vi "TreeSelectBratCallback.vi"(4 "Glyph Indices":T1, 5 "Event Data":T3, 6 "Tree Ref":refnum<vi>, 7 "Event Common Data":cluster{"Source":T4, "Type":T5, "Time":u32} {"Source" items=["LabVIEW UI"=0, "ActiveX"=1, "User Event"=25]}) -> ()   [LabVIEW 2012]
uses:
  <vilib>/event_ctls.llb/eventsource.ctl
  <vilib>/event_ctls.llb/lveventtype.ctl
  <vilib>/Utility/miscctls.llb/LVPoint32TypeDef.ctl
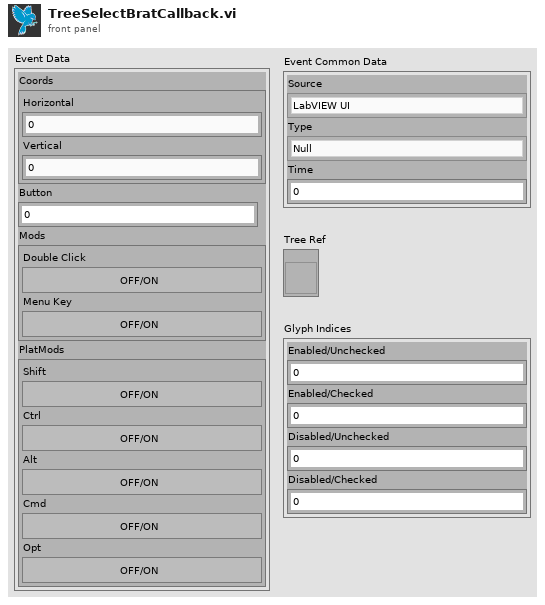
[diagram p1: front panel]
types:
  T1 = cluster{"Enabled/Unchecked":i32, "Enabled/Checked":i32, "Disabled/Unchecked":i32, "Disabled/Checked":i32}
  T2 = typedef "LVPoint32TypeDef.ctl" = cluster{"Horizontal":i32, "Vertical":i32}
  T3 = cluster{"Coords":T2, "Button":u16, "Mods":cluster{"Double Click":bool, "Menu Key":bool}, "PlatMods":cluster{"Shift":bool, "Ctrl":bool, "Alt":bool, "Cmd":bool, "Opt":bool}}
  T4 = typedef "eventsource.ctl" = u32
  T5 = typedef "lveventtype.ctl" = enum32{"Null", "Timeout", "Annotation Menu Selection", "Annotation Menu Selection?", "App Instance Close", "App Instance Close?", "Autoscale Range Change", "Cell Edit", "Cell Edit?", "Cursor Grab", "Cursor Grab?", "Cursor Menu Selection", "Cursor Menu Selection?", "Cursor Move", "Cursor Release", "Data Change", "Direction Change", "Display State Change", "Drag Ended", "Drag Enter", "Drag Leave", "Drag Over", "Drag Source Update", "Drag Starting", "Drag Starting?", "Drop", "Exec State Change", "Key Down", "Key Down?", "Key Repeat", "Key Repeat?", "Key Up", "Listbox Double Click", "Menu Activation?", "Menu Selection (App)", "Menu Selection? (App)", "Menu Selection (User)", "Mouse Down", "Mouse Down?", "Mouse Enter", "Mouse Leave", "Mouse Move", "Mouse Up", "NI Security User Change (App)", "Pane Size", "Panel Close", "Panel Close?", "Panel Resize", "Plot Attribute Change", "Scale Range Change", "Shortcut Menu Activation?", "Shortcut Menu Selection (App)", "Shortcut Menu Selection? (App)", "Shortcut Menu Selection (User)", "Tree Double Click", "Tree Drag", "Tree Drag?", "Tree Drop", "Tree Drop?", "Tree Item Close", "Tree Item Close?", "Tree Item Open", "Tree Item Open?", "Value Change"}
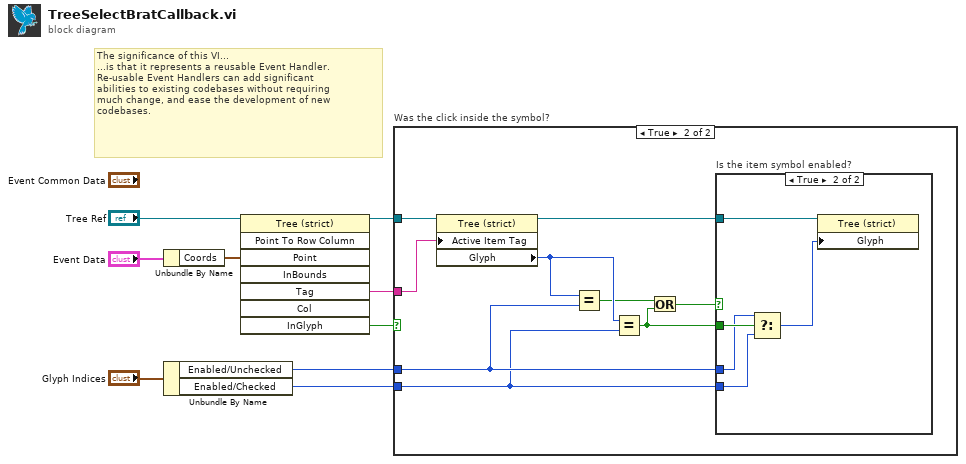
[diagram p0: block diagram]
diagram:
  # "The significance of this VI...\n...is that it represents a reusable Event Handler.\nRe-usable Event Handlers can add significant\nabilities to existing codebases without requiring\nmuch change, and ease the development of new\ncodebases."
  n1 = Unbundle By Name("Event Data") -> ("Coords"=w7:T2)
  n2 = Unbundle By Name("Glyph Indices") -> ("Enabled/Unchecked"=w3:i32, "Enabled/Checked"=w1:i32)
  n3 = invoke class="Tree (strict)" method="Point To Row Column"(reference="Tree Ref", "Point"=w7) -> (reference out=w6:refnum<vi>, "Tag"=w5:string, "InGlyph"=w2:bool)  [unwired: 6 in, 5 out]
  n4 = case "Was the click inside the symbol?" shown="True" w2 {
    tunnel: w6 -> [_ w18]
    tunnel: w5 -> [_ w17]
    tunnel: w3 -> [_ w13]
    tunnel: w1 -> [_ w11]
    frame False {
    }
    frame True {
      n5 = property class="Tree (strict)"(reference=w18, "Active Item Tag"=w17) -> (reference out=w15:refnum<vi>, "Glyph"=w16:i32)  [unwired: 1 in, 1 out]
      n6 = Equal?(x=w16, y=w13) -> (x = y?=w12:bool)
      n7 = Equal?(x=w16, y=w11) -> (x = y?=w10:bool)
      n8 = Or(x=w12, y=w10) -> (x .or. y?=w14:bool)
      n9 = case "Is the item symbol enabled?" shown="True" w14 {
        tunnel: w15 -> [_ w23]
        tunnel: w13 -> [_ w21]
        tunnel: w11 -> [_ w20]
        tunnel: w10 -> [_ w22]
        frame False {
        }
        frame True {
          n10 = Select(t=w21, s=w22, f=w20) -> (s? t:f=w19:i32)
          n11 = property class="Tree (strict)"(reference=w23, "Glyph"=w19) -> ()  [unwired: 1 in, 2 out]
        }
      }
    }
  }
